vi "Check Valid Type.vi"(9 "Requested type":T1=enum."type", 10 "Item type":string) -> (2 "Valid?":bool)   [LabVIEW 2013, in "CConfig Object.lvclass"]
doc: "Copyright 2018, Carya Automatisering, Wiebe Walstra."
uses:
  CConfig Object.lvclass
  Data.ctl
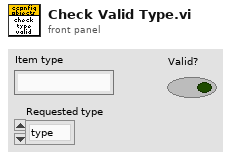
[diagram p1: front panel]
types:
  T1 = typedef "CConfig Object.lvclass/Data.ctl" = enum16{"pre", "name", "middle", "value", "post", "newline", "persistant", "tagged", "type"}
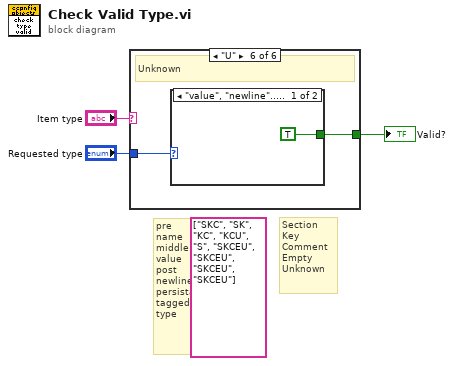
[diagram p0: block diagram]
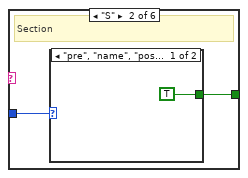
[diagram p3: hidden frame]
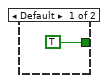
[diagram p6: hidden frame]
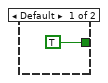
[diagram p8: hidden frame]
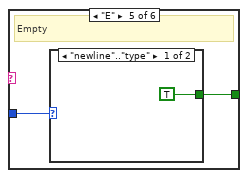
[diagram p9: hidden frame]
diagram:
  (unwired) string[] ["SKC", "SK", "KC", "KCU", "S", "SKCEU", "SKCEU", "SKCEU", "SKCEU"]
  # "pre\nname\nmiddle\nvalue\npost \nnewline\npersistant\ntagged\ntype"
  # "Section\nKey\nComment\nEmpty\nUnknown"
  n1 = case shown="\"U\"" "Item type" {
    tunnel: "Requested type" -> [_ w5 w8 w11 w14 w17]
    tunnel: [_ w4 w7 w10 w13 w16] -> w1
    frame Default {
    }
    frame "S" {
      # "Section"
      n2 = case shown="\"pre\", \"name\", \"post\"..\"type\"" w5 {
        tunnel: [TRUE _] -> w4
        frame "pre", "name", "post".."type" {
        }
        frame Default {
        }
      }
    }
    frame "K" {
      # "Key"
      n3 = case shown="\"post\"" w8 {
        tunnel: [TRUE _] -> w7
        frame Default {
        }
        frame "post" {
        }
      }
    }
    frame "C" {
      # "Comment"
      n4 = case shown="\"name\", \"post\"" w11 {
        tunnel: [TRUE _] -> w10
        frame Default {
        }
        frame "name", "post" {
        }
      }
    }
    frame "E" {
      # "Empty"
      n5 = case shown="\"newline\"..\"type\"" w14 {
        tunnel: [TRUE _] -> w13
        frame "newline".."type" {
        }
        frame Default {
        }
      }
    }
    frame "U" {
      # "Unknown"
      n6 = case shown="\"value\", \"newline\"..\"type\"" w17 {
        tunnel: [TRUE _] -> w16
        frame "value", "newline".."type" {
        }
        frame Default {
        }
      }
    }
  }
  "Valid?" <- w1
